vi "Ophir StringToValue.vi"(2 "error in (no error)":errorcluster, 3 "Frame":string) -> (0 "error out":errorcluster, 1 "Value":dbl format="%.3e")   [LabVIEW 2017]
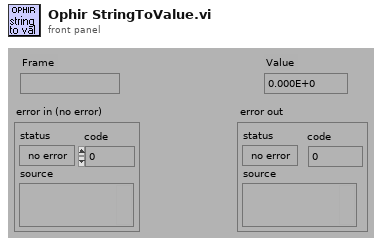
[diagram p1: front panel]
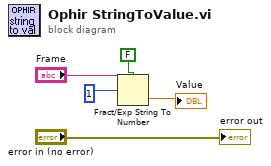
[diagram p0: block diagram]
diagram:
  n1 = Fract/Exp String To Number(use system decimal point (T)=FALSE, string="Frame", offset=1) -> (number=→"Value":dbl)  [unwired: 2 out]
  "error out" <- "error in (no error)"
